vi "XML_MatchPatten.vi"(6 "first(T)/Last(F)":bool, 8 "offset (0)":i32, 10 "tag":string, 11 "XML":T1) -> (0 "offset past match":i32, 1 "after substring":T1, 2 "concatenated string out":T1, 3 "before substring":T1)   [LabVIEW 2017]
doc: "Splits XML at the first or last occurrence of the element named by tag, starting the search at offset, and returns the text before and after the match together with the offset past it."
uses:
  _XML--String.ctl
  <vilib>/regexp/Match Regular Expression.xnode
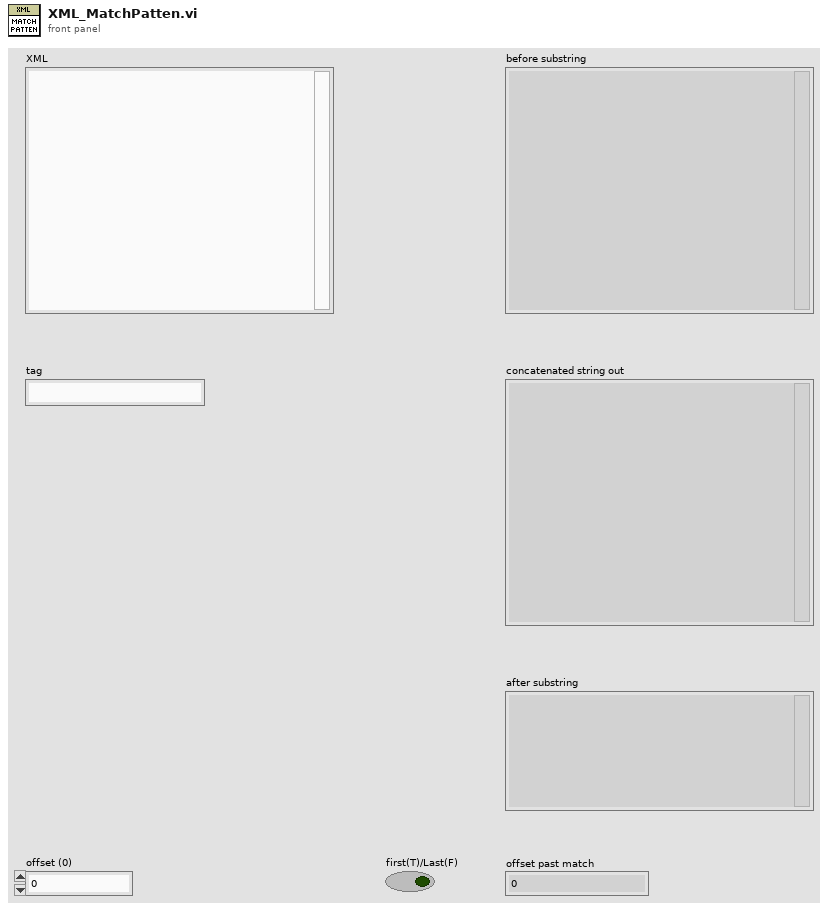
[diagram p1: front panel]
types:
  T1 = typedef "_XML--String.ctl" = string
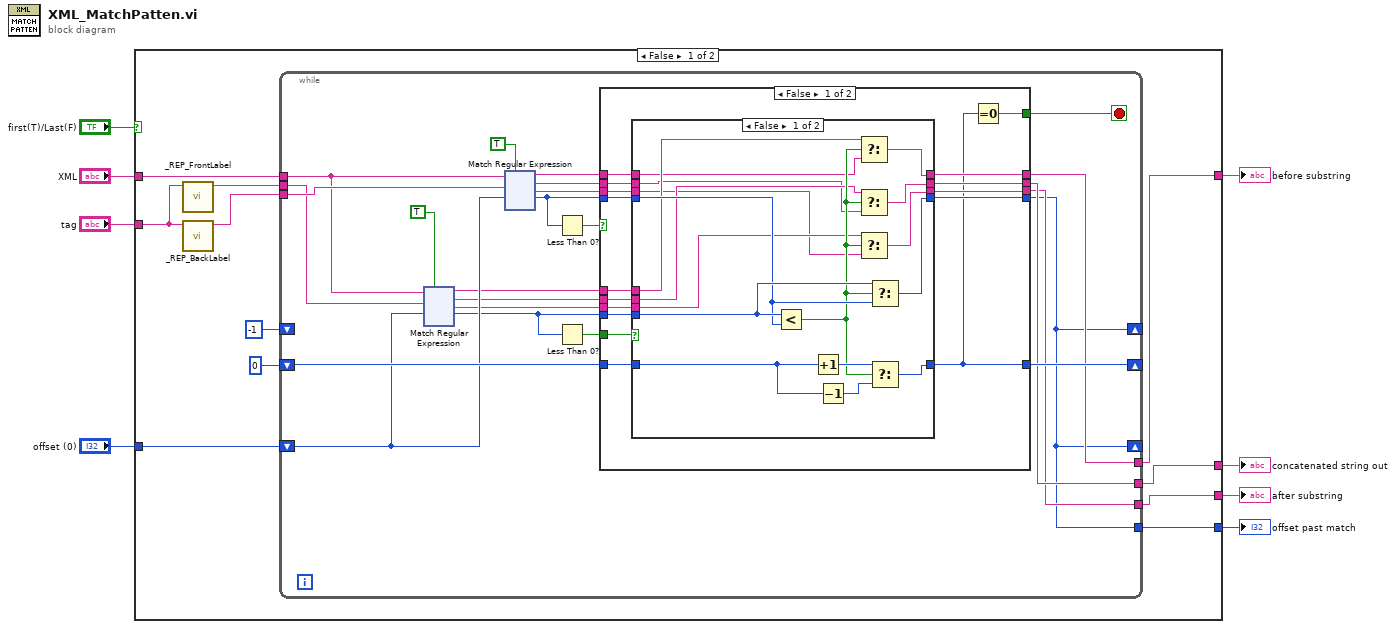
[diagram p0: block diagram]
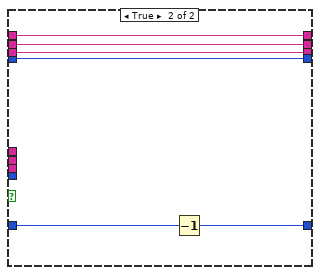
[diagram p2: hidden frame]
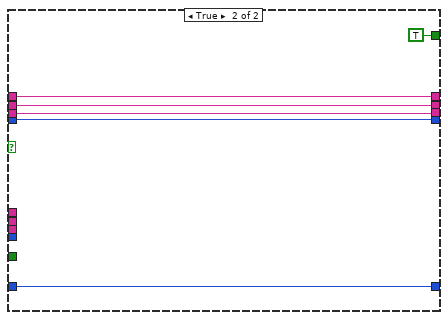
[diagram p3: hidden frame]
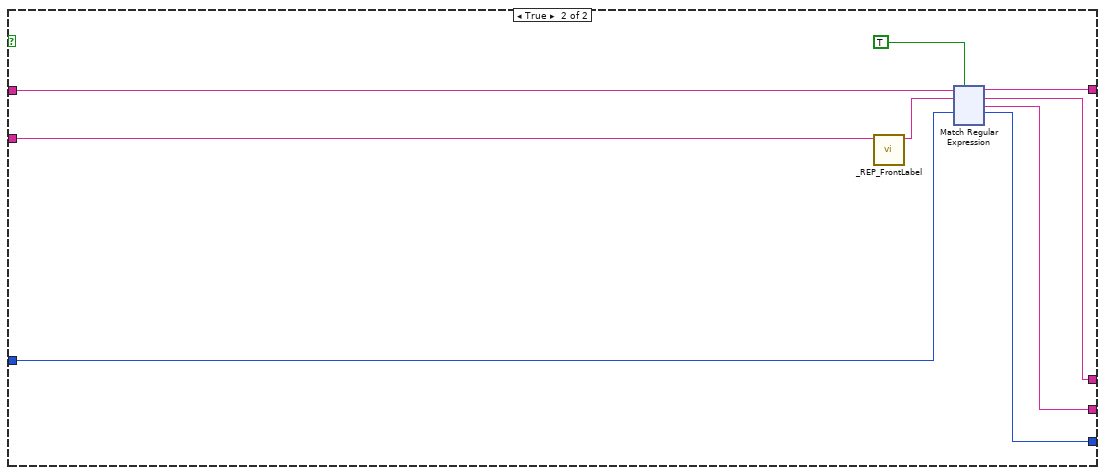
[diagram p4: hidden frame]
diagram:
  n1 = case shown="False" "first(T)/Last(F)" {
    tunnel: "XML" -> [w19 w320]
    tunnel: "tag" -> [w14 w317]
    tunnel: [w10 w324] -> w6
    tunnel: [w17 w318] -> w5
    tunnel: "offset (0)" -> [w18 w323]
    tunnel: [w11 w322] -> w3
    tunnel: [w9 w321] -> w2
    frame False {
      n2 = call "_REP_FrontLabel.vi"("label"=w14) -> ("String"=w13:string)  [unwired: 10 in]
      n3 = call "_REP_BackLabel.vi"("label"=w14) -> ("String"=w15:string)  [unwired: 10 in]
      n4 = while {
        tunnel: w19 -> [w39]
        tunnel: w15 -> [w42]
        shift-right: [w20] -> _
        shift-left: w18 -> [w36]
        tunnel: [w20] -> w17
        shift-right: [w20] -> _
        shift-left: -1 ("t") -> [_]
        tunnel: w13 -> [w38]
        shift-right: [w32] -> _
        shift-left: 0 ("t") -> [w37]
        tunnel: [w29] -> w11
        tunnel: [w26] -> w10
        tunnel: [w24] -> w9
        stop <- w30 stop-if-true
        n5 = xnode "Match Regular Expression"("input string"=w39, "regular expression"=w38, "offset (0)"=w36, "ignore case? (F)"=TRUE) -> ("before match"=w23:string, "whole match"=w22:string, "after match"=w21:string, "offset past match"=w34:i32)  [unwired: 2 in, 1 out]
        n6 = xnode "Match Regular Expression"("input string"=w39, "regular expression"=w42, "offset (0)"=w36, "ignore case? (F)"=TRUE) -> ("before match"=w28:string, "whole match"=w27:string, "after match"=w25:string, "offset past match"=w35:i32)  [unwired: 2 in, 1 out]
        n7 = Less Than 0?(x=w35) -> (x < 0?=w31:bool)
        n8 = Less Than 0?(x=w34) -> (x < 0?=w33:bool)
        n9 = case shown="False" w31 {
          tunnel: w37 -> [w58 w87]
          tunnel: w35 -> [w57 w85]
          tunnel: w34 -> [w56 _]
          tunnel: w33 -> [w55 _]
          tunnel: [w43 w87] -> w32
          tunnel: [w54 TRUE] -> w30
          tunnel: [w44 w85] -> w20
          tunnel: [w47 w84] -> w29
          tunnel: w28 -> [w53 w84]
          tunnel: w27 -> [w52 w83]
          tunnel: [w46 w83] -> w26
          tunnel: w25 -> [w51 w82]
          tunnel: [w45 w82] -> w24
          tunnel: w23 -> [w50 _]
          tunnel: w22 -> [w49 _]
          tunnel: w21 -> [w48 _]
          frame False {
            n10 = case shown="False" w55 {
              tunnel: w56 -> [w70 _]
              tunnel: w57 -> [w69 w76]
              tunnel: w58 -> [w75 w81]
              tunnel: [w72 w80] -> w43
              tunnel: w53 -> [w62 w79]
              tunnel: w52 -> [w63 w78]
              tunnel: w51 -> [w64 w77]
              tunnel: w50 -> [w67 _]
              tunnel: w49 -> [w66 _]
              tunnel: w48 -> [w65 _]
              tunnel: [w61 w79] -> w47
              tunnel: [w60 w78] -> w46
              tunnel: [w59 w77] -> w45
              tunnel: [w71 w76] -> w44
              frame False {
                n11 = Less?(x=w70, y=w69) -> (x < y?=w68:bool)
                n12 = Increment(x=w75) -> (x+1=w74:i32)
                n13 = Decrement(x=w75) -> (x-1=w73:i32)
                n14 = Select(t=w67, s=w68, f=w62) -> (s? t:f=w61:string)
                n15 = Select(t=w66, s=w68, f=w63) -> (s? t:f=w60:string)
                n16 = Select(t=w65, s=w68, f=w64) -> (s? t:f=w59:string)
                n17 = Select(t=w70, s=w68, f=w69) -> (s? t:f=w71:i32)
                n18 = Select(t=w74, s=w68, f=w73) -> (s? t:f=w72:i32)
              }
              frame True {
                n19 = Decrement(x=w81) -> (x-1=w80:i32)
              }
            }
            n20 = Equal To 0?(x=w43) -> (x = 0?=w54:bool)
          }
          frame True {
          }
        }
      }
    }
    frame True {
      n21 = call "_REP_FrontLabel.vi"("label"=w317) -> ("String"=w316:string)  [unwired: 10 in]
      n22 = xnode "Match Regular Expression"("input string"=w320, "regular expression"=w316, "offset (0)"=w323, "ignore case? (F)"=TRUE) -> ("before match"=w322:string, "whole match"=w324:string, "after match"=w321:string, "offset past match"=w318:i32)  [unwired: 2 in, 1 out]
    }
  }
  "concatenated string out" <- w6
  "offset past match" <- w5
  "before substring" <- w3
  "after substring" <- w2
